vi "AutoRun.vi"() -> ()   [LabVIEW 2012]
uses:
  resultShow.vi
panel:
  in  "布尔":bool
  out "毫秒计时值":u32
  in  "stepMotor/ECU":string
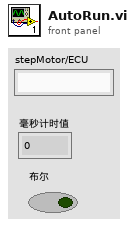
[diagram p1: front panel]
types:
  T1 = cluster{"takesTime":refnum<vi>, "userStatus":refnum<vi>, "userName":refnum<vi>, "connectionMode":refnum<vi>, "productsName":refnum<vi>, "rigStatus":refnum<vi>, "管柱码":refnum<vi>}
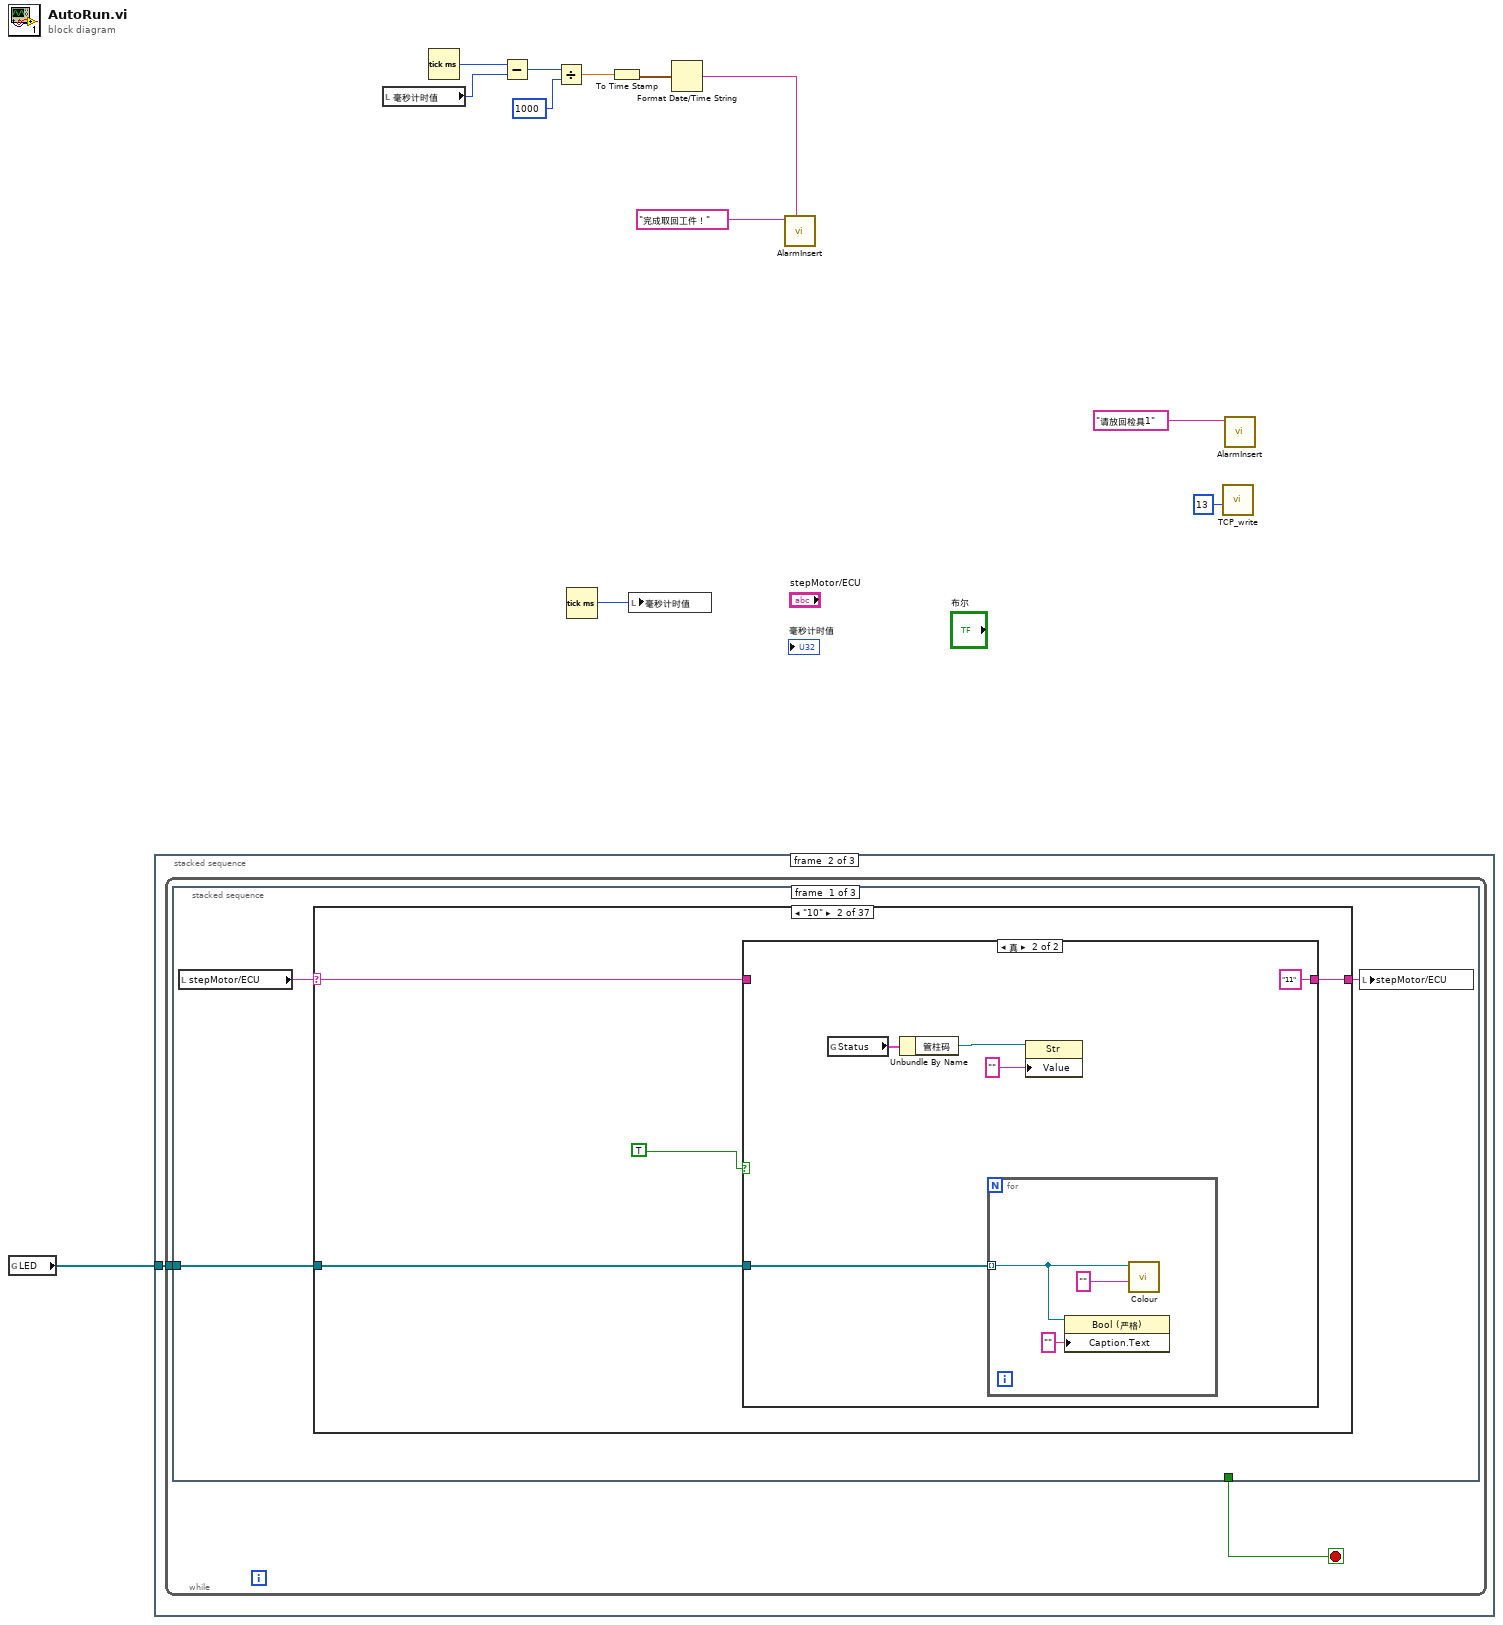
[diagram p0: block diagram]
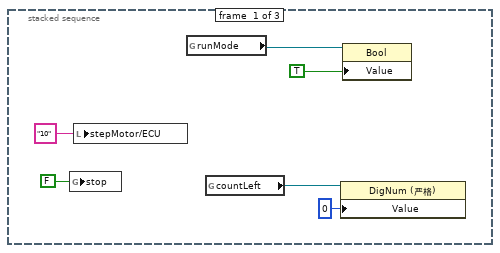
[diagram p2: hidden frame]
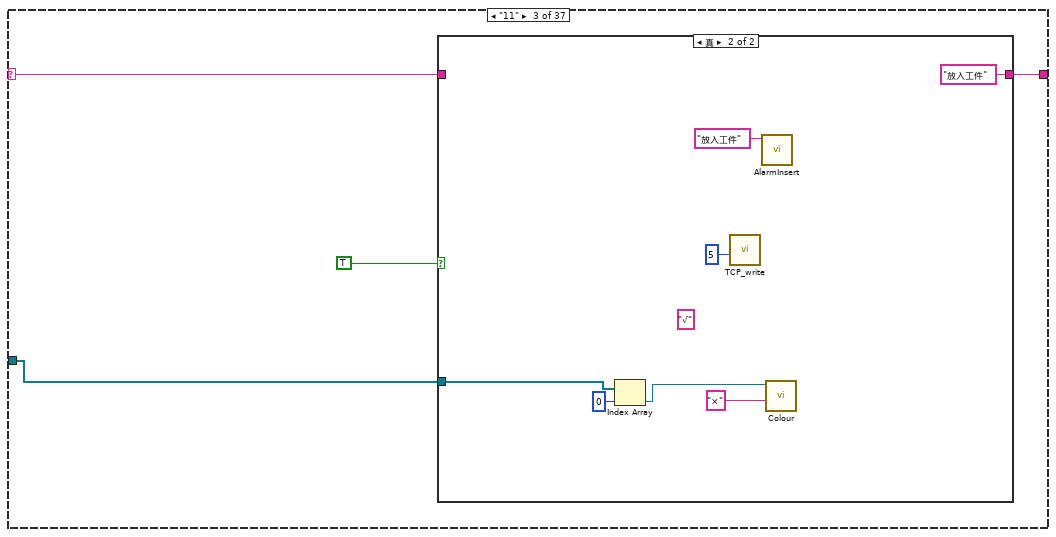
[diagram p5: hidden frame]
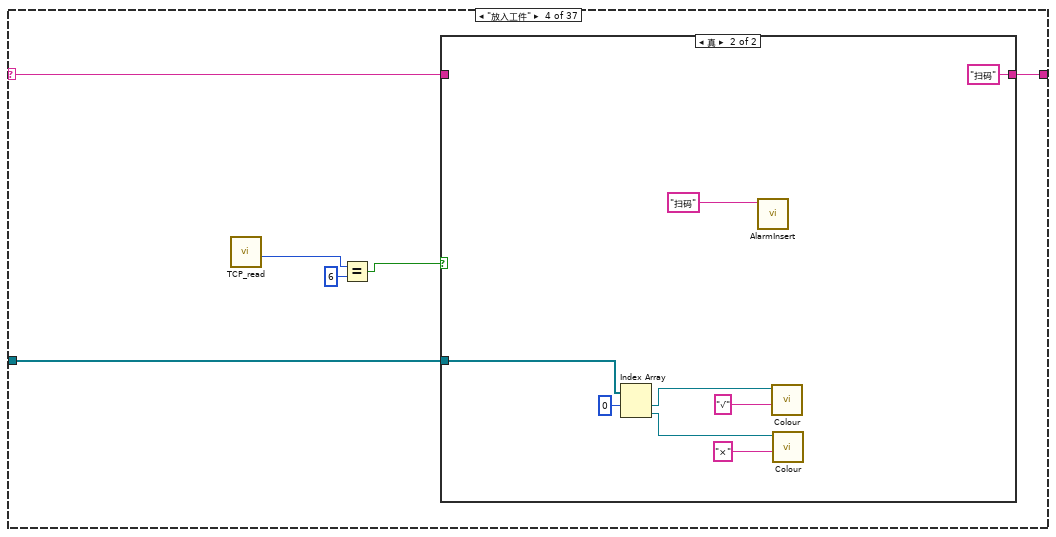
[diagram p7: hidden frame]
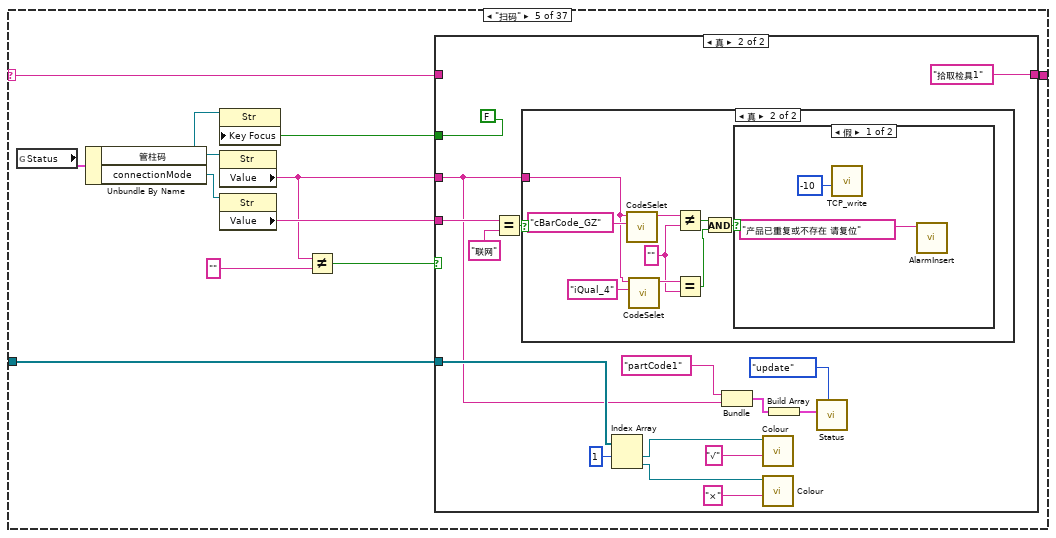
[diagram p9: hidden frame]
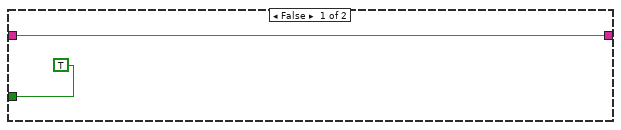
[diagram p10: hidden frame]
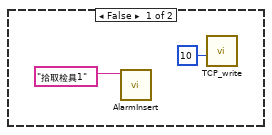
[diagram p11: hidden frame]
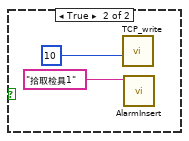
[diagram p12: hidden frame]
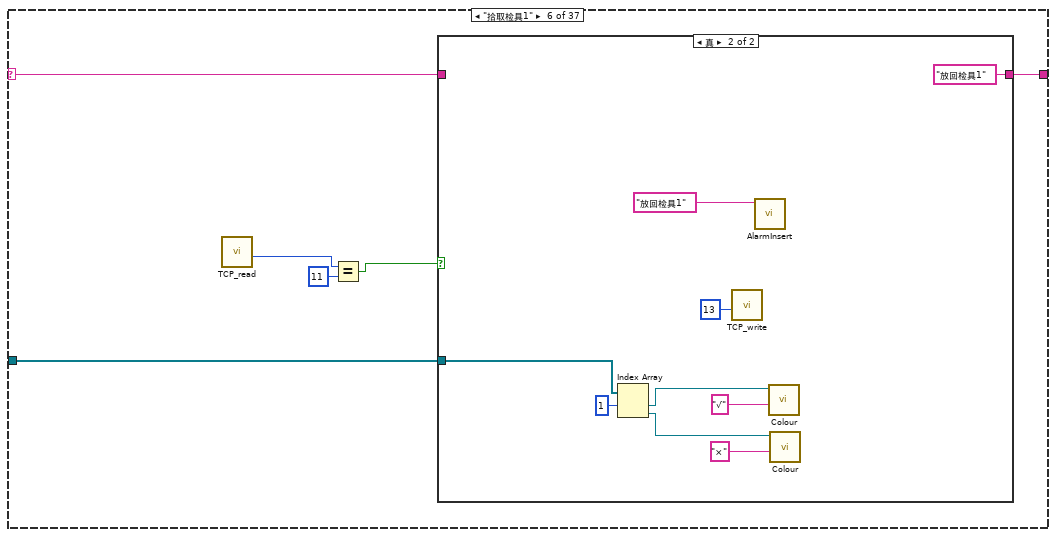
[diagram p13: hidden frame]
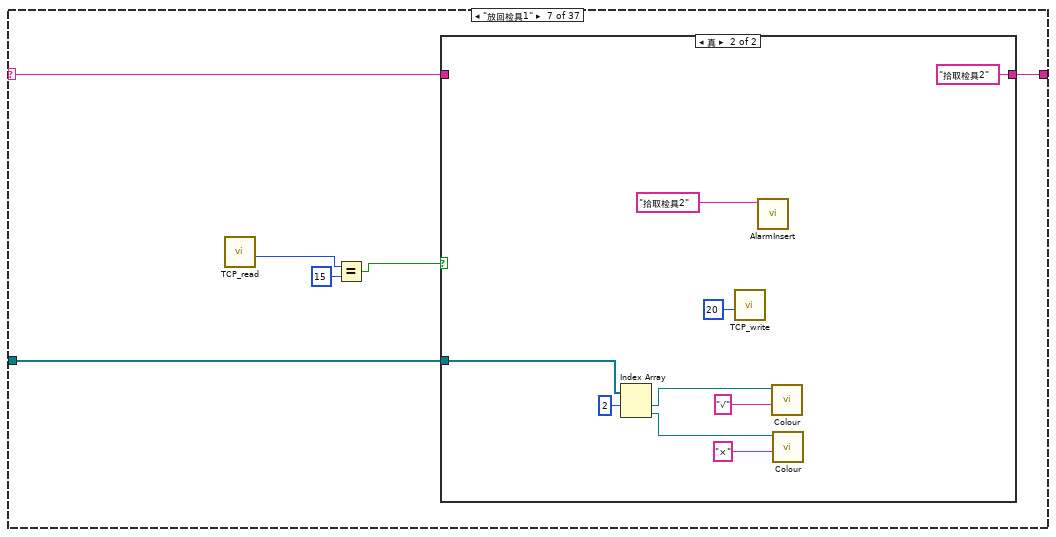
[diagram p15: hidden frame]
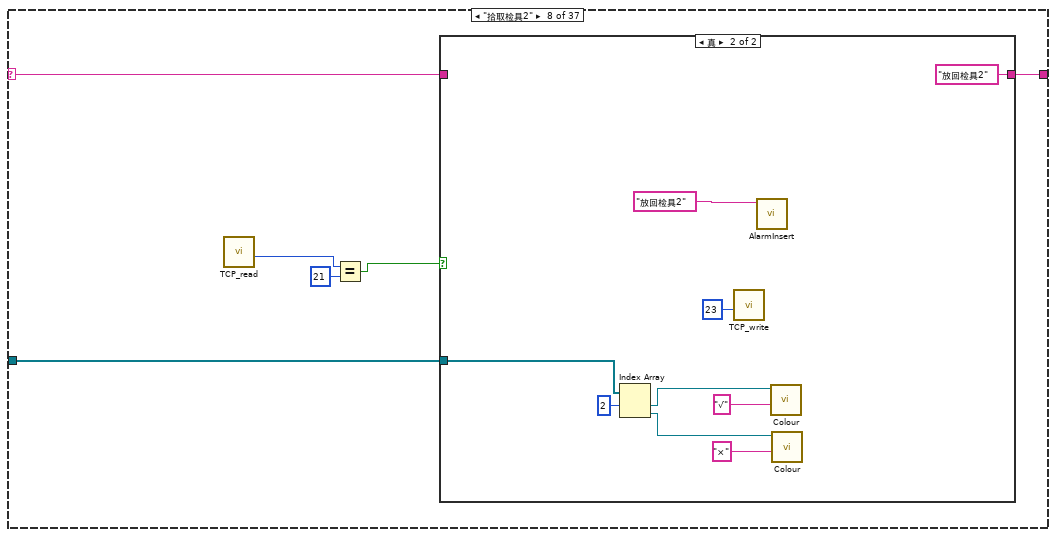
[diagram p17: hidden frame]
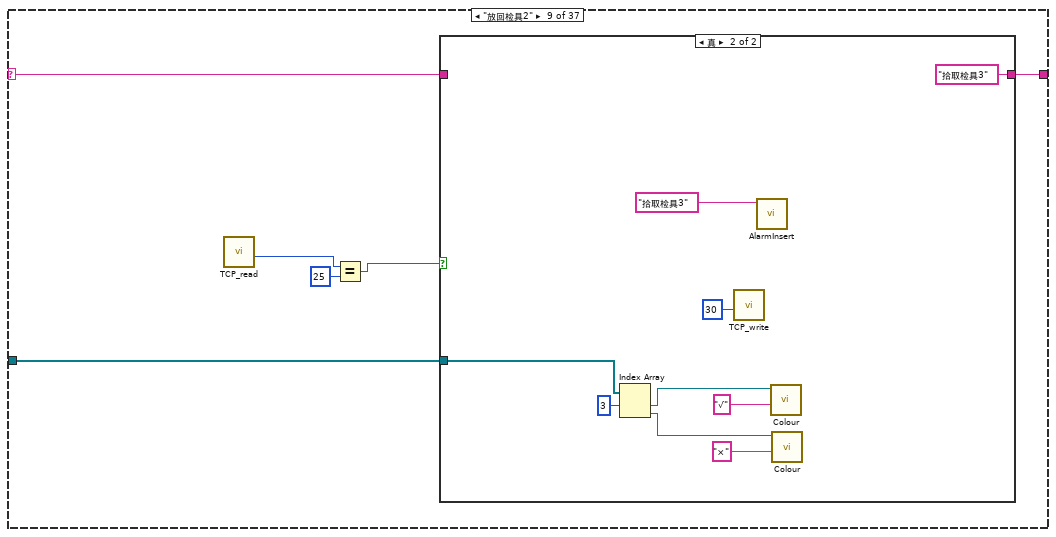
[diagram p19: hidden frame]
diagram:
  n1 = global read "resultShow.vi" "LED"() -> (w12:refnum<vi>[])
  n2 = stacked-sequence {
    tunnel: w12 -> [_ w19 _]
    frame #0 {
      n3 = global write "全局 3.vi" "stop"(FALSE ("布尔 2")) -> ()
      n4 = local write "stepMotor/ECU"("10" ("step")) -> ()
      n5 = global read "resultShow.vi" "runMode"() -> (w15:refnum<vi>)
      n6 = global read "resultShow.vi" "countLeft"() -> (w13:refnum<vi>)
      n7 = property class="DigNum (严格)"(reference=w13, "Value"=u32 0 ("值")) -> ()  [unwired: 1 in, 2 out]
      n8 = property class="Bool"(reference=w15, "Value"=TRUE ("m")) -> ()  [unwired: 1 in, 2 out]
    }
    frame #1 {
      n9 = while {
        tunnel: w19 -> [w20]
        stop <- w21 stop-if-true
        n10 = stacked-sequence {
          tunnel: [_ _ w657] -> w21
          tunnel: w20 -> [w23 _ _]
          frame #0 {
            n11 = local read "stepMotor/ECU"() -> (w22:string)
            n12 = case shown="\"10\"" w22 {
              selector: w22 -> [w25 w28 w41 w53 w75 w114 w128 w144 w160 w178 w194 w210 w226 w242 w258 w274 w290 w306 w322 w338 w354 w370 w386 w402 w418 w434 w450 w466 w482 w498 w514 w530 w546 w562 w578 w592 w620]
              tunnel: [w25 w29 w42 w51 w74 w115 w126 w142 w158 w179 w195 w211 w227 w243 w259 w275 w291 w307 w323 w339 w355 w371 w387 w403 w419 w435 w451 w467 w483 w499 w515 w531 w547 w563 w579 w593 w621] -> w24
              tunnel: w23 -> [_ w27 w40 w52 w76 w110 w127 w143 w159 w174 w190 w206 w222 w238 w254 w270 w286 w302 w318 w334 w350 w366 w382 w398 w414 w430 w446 w462 w478 w494 w510 w526 w542 w558 w574 w591 w616]
              frame "假", Default {
              }
              frame "10" {
                n13 = case shown="真" TRUE {
                  tunnel: [w30 "11"] -> w29
                  tunnel: w28 -> [w30 _]
                  tunnel: w27 -> [_ w34]
                  frame False {
                  }
                  frame True {
                    n14 = global read "resultShow.vi" "Status"() -> (w32:T1)
                    n15 = Unbundle By Name(w32) -> ("管柱码"=w31:refnum<vi>)
                    n16 = for {
                      tunnel: w34 -> [w37] mode=indexing
                      n17 = property class="Bool (严格)"(reference=w37, "Caption.Text"="" ("标题.文本")) -> ()  [unwired: 1 in, 2 out]
                      n18 = call "Colour.vi"("result"="" ("元素"), "colourRef"=w37) -> ()  [unwired: 9 in, 1 out]
                    }
                    n19 = property class="Str"(reference=w31, "Value"="") -> ()  [unwired: 1 in, 2 out]
                  }
                }
              }
              frame "11" {
                n20 = case shown="真" TRUE {
                  tunnel: [w43 "放入工件"] -> w42
                  tunnel: w41 -> [w43 _]
                  tunnel: w40 -> [_ w46]
                  frame False {
                  }
                  frame True {
                    (unwired) "√" ("元素")
                    n21 = Index Array(array=w46, index=0 ("索引")) -> (element=w48:refnum<vi>)
                    n22 = call "TCP_write.vi"("写入数据"=i8 5) -> ()  [unwired: 11 in]
                    n23 = call "AlarmInsert.vi"("消息名"="放入工件") -> ()  [unwired: 11 in]
                    n24 = call "Colour.vi"("result"="×" ("元素"), "colourRef"=w48) -> ()  [unwired: 9 in, 1 out]
                  }
                }
              }
              frame "放入工件" {
                n25 = call "TCP_read.vi"() -> ("元素"=w54:i8)  [unwired: 10 in, 1 out]
                n26 = Equal?(x=w54, y=i8 6) -> (x = y?=w56:bool)
                n27 = case shown="真" w56 {
                  tunnel: [w57 "扫码"] -> w51
                  tunnel: w53 -> [w57 _]
                  tunnel: w52 -> [_ w59]
                  frame False {
                  }
                  frame True {
                    n28 = Index Array(array=w59, index #1=0 ("索引")) -> (element #1=w63:refnum<vi>, element #2=w60:refnum<vi>)  [unwired: 1 in]
                    n29 = call "AlarmInsert.vi"("消息名"="扫码" ("string_5")) -> ()  [unwired: 11 in]
                    n30 = call "Colour.vi"("result"="√" ("元素"), "colourRef"=w63) -> ()  [unwired: 9 in, 1 out]
                    n31 = call "Colour.vi"("result"="×" ("元素"), "colourRef"=w60) -> ()  [unwired: 9 in, 1 out]
                  }
                }
              }
              frame "扫码" {
                n32 = global read "resultShow.vi" "Status"() -> (w73:T1)
                n33 = Unbundle By Name(w73) -> ("管柱码"=w71:refnum<vi>, "connectionMode"=w68:refnum<vi>)
                n34 = property class="Str"(reference=w71) -> ("Value"=w66:string)  [unwired: 1 in, 2 out]
                n35 = property class="Str"(reference=w68) -> ("Value"=w67:string)  [unwired: 1 in, 2 out]
                n36 = Not Equal?(x=w66, y="") -> (x != y?=w70:bool)
                n37 = case shown="真" w70 {
                  tunnel: [w78 "拾取检具1"] -> w74
                  tunnel: w75 -> [w78 _]
                  tunnel: w76 -> [_ w90]
                  tunnel: [TRUE FALSE] -> w69
                  tunnel: w67 -> [_ w85]
                  tunnel: w66 -> [_ w81]
                  frame False {
                  }
                  frame True {
                    n38 = Equal?(x=w85, y="联网") -> (x = y?=w84:bool)
                    n39 = case shown="真" w84 {
                      tunnel: w81 -> [_ w100]
                      frame False {
                        n40 = call "AlarmInsert.vi"("消息名"="拾取检具1") -> ()  [unwired: 11 in]
                        n41 = call "TCP_write.vi"("写入数据"=i8 10) -> ()  [unwired: 11 in]
                      }
                      frame True {
                        w97 = "" ("元素")
                        n42 = call "CodeSelet.vi"("字符串"="cBarCode_GZ" ("code"), "parameter name"=w100) -> ("readData"=w102:string)  [unwired: 9 in]
                        n43 = call "CodeSelet.vi"("字符串"="iQual_4" ("code"), "parameter name"=w100) -> ("readData"=w99:string)  [unwired: 9 in]
                        n44 = Not Equal?(x=w102, y=w97) -> (x != y?=w105:bool)
                        n45 = Equal?(x=w99, y=w97) -> (x = y?=w104:bool)
                        n46 = And(x=w105, y=w104) -> (x .and. y?=w103:bool)
                        n47 = case shown="假" w103 {
                          frame False {
                            n48 = call "TCP_write.vi"("写入数据"=i8 -10) -> ()  [unwired: 11 in]
                            n49 = call "AlarmInsert.vi"("消息名"="产品已重复或不存在 请复位") -> ()  [unwired: 11 in]
                          }
                          frame True {
                            n50 = call "TCP_write.vi"("写入数据"=i8 10) -> ()  [unwired: 11 in]
                            n51 = call "AlarmInsert.vi"("消息名"="拾取检具1") -> ()  [unwired: 11 in]
                          }
                        }
                      }
                    }
                    n52 = Index Array(array=w90, index #1=1 ("索引")) -> (element #1=w92:refnum<vi>, element #2=w88:refnum<vi>)  [unwired: 1 in]
                    n53 = Bundle("元素"="partCode1", "Value"=w81) -> (w83:cluster{"元素":string, "Value":string})  [unwired: 1 in]
                    n54 = call "Colour.vi"("result"="√" ("元素"), "colourRef"=w92) -> ()  [unwired: 9 in, 1 out]
                    n55 = call "Colour.vi"("result"="×" ("元素"), "colourRef"=w88) -> ()  [unwired: 9 in, 1 out]
                    n56 = Build Array(w83) -> (w80:cluster{"元素":string, "Value":string}[])
                    n57 = call "Status.vi"("模式"=enum16{"select", "insert", "update", "delete"}."update", "nameData"=w80) -> ()  [unwired: 9 in, 1 out]
                  }
                }
                n58 = property class="Str"(reference=w71, "Key Focus"=w69) -> ()  [unwired: 1 in, 2 out]
              }
              frame "拾取检具1" {
                n59 = call "TCP_read.vi"() -> ("元素"=w113:i8)  [unwired: 10 in, 1 out]
                n60 = Equal?(x=w113, y=i8 11) -> (x = y?=w111:bool)
                n61 = case shown="真" w111 {
                  tunnel: [w116 "放回检具1"] -> w115
                  tunnel: w114 -> [w116 _]
                  tunnel: w110 -> [_ w118]
                  frame False {
                  }
                  frame True {
                    n62 = Index Array(array=w118, index #1=1 ("索引")) -> (element #1=w122:refnum<vi>, element #2=w119:refnum<vi>)  [unwired: 1 in]
                    n63 = call "TCP_write.vi"("写入数据"=i8 13) -> ()  [unwired: 11 in]
                    n64 = call "AlarmInsert.vi"("消息名"="放回检具1" ("string_5")) -> ()  [unwired: 11 in]
                    n65 = call "Colour.vi"("result"="√" ("元素"), "colourRef"=w122) -> ()  [unwired: 9 in, 1 out]
                    n66 = call "Colour.vi"("result"="×" ("元素"), "colourRef"=w119) -> ()  [unwired: 9 in, 1 out]
                  }
                }
              }
              frame "放回检具1" {
                n67 = call "TCP_read.vi"() -> ("元素"=w131:i8)  [unwired: 10 in, 1 out]
                n68 = Equal?(x=w131, y=i8 15) -> (x = y?=w129:bool)
                n69 = case shown="真" w129 {
                  tunnel: [w132 "拾取检具2"] -> w126
                  tunnel: w128 -> [w132 _]
                  tunnel: w127 -> [_ w134]
                  frame False {
                  }
                  frame True {
                    n70 = Index Array(array=w134, index #1=2 ("索引")) -> (element #1=w138:refnum<vi>, element #2=w135:refnum<vi>)  [unwired: 1 in]
                    n71 = call "TCP_write.vi"("写入数据"=i8 20) -> ()  [unwired: 11 in]
                    n72 = call "AlarmInsert.vi"("消息名"="拾取检具2" ("string_5")) -> ()  [unwired: 11 in]
                    n73 = call "Colour.vi"("result"="√" ("元素"), "colourRef"=w138) -> ()  [unwired: 9 in, 1 out]
                    n74 = call "Colour.vi"("result"="×" ("元素"), "colourRef"=w135) -> ()  [unwired: 9 in, 1 out]
                  }
                }
              }
              frame "拾取检具2" {
                n75 = call "TCP_read.vi"() -> ("元素"=w145:i8)  [unwired: 10 in, 1 out]
                n76 = Equal?(x=w145, y=i8 21) -> (x = y?=w147:bool)
                n77 = case shown="真" w147 {
                  tunnel: [w148 "放回检具2"] -> w142
                  tunnel: w144 -> [w148 _]
                  tunnel: w143 -> [_ w150]
                  frame False {
                  }
                  frame True {
                    n78 = Index Array(array=w150, index #1=2 ("索引")) -> (element #1=w154:refnum<vi>, element #2=w151:refnum<vi>)  [unwired: 1 in]
                    n79 = call "TCP_write.vi"("写入数据"=i8 23) -> ()  [unwired: 11 in]
                    n80 = call "AlarmInsert.vi"("消息名"="放回检具2" ("string_5")) -> ()  [unwired: 11 in]
                    n81 = call "Colour.vi"("result"="√" ("元素"), "colourRef"=w154) -> ()  [unwired: 9 in, 1 out]
                    n82 = call "Colour.vi"("result"="×" ("元素"), "colourRef"=w151) -> ()  [unwired: 9 in, 1 out]
                  }
                }
              }
              frame "放回检具2" {
                n83 = call "TCP_read.vi"() -> ("元素"=w161:i8)  [unwired: 10 in, 1 out]
                n84 = Equal?(x=w161, y=i8 25) -> (x = y?=w163:bool)
                n85 = case shown="真" w163 {
                  tunnel: [w164 "拾取检具3"] -> w158
                  tunnel: w160 -> [w164 _]
                  tunnel: w159 -> [_ w166]
                  frame False {
                  }
                  frame True {
                    n86 = Index Array(array=w166, index #1=3 ("索引")) -> (element #1=w170:refnum<vi>, element #2=w167:refnum<vi>)  [unwired: 1 in]
                    n87 = call "TCP_write.vi"("写入数据"=i8 30) -> ()  [unwired: 11 in]
                    n88 = call "AlarmInsert.vi"("消息名"="拾取检具3" ("string_5")) -> ()  [unwired: 11 in]
                    n89 = call "Colour.vi"("result"="√" ("元素"), "colourRef"=w170) -> ()  [unwired: 9 in, 1 out]
                    n90 = call "Colour.vi"("result"="×" ("元素"), "colourRef"=w167) -> ()  [unwired: 9 in, 1 out]
                  }
                }
              }
              frame "拾取检具3" {
                n91 = call "TCP_read.vi"() -> ("元素"=w177:i8)  [unwired: 10 in, 1 out]
                n92 = Equal?(x=w177, y=i8 31) -> (x = y?=w175:bool)
                n93 = case shown="真" w175 {
                  tunnel: [w180 "放回检具3"] -> w179
                  tunnel: w178 -> [w180 _]
                  tunnel: w174 -> [_ w182]
                  frame False {
                  }
                  frame True {
                    n94 = Index Array(array=w182, index #1=3 ("索引")) -> (element #1=w186:refnum<vi>, element #2=w183:refnum<vi>)  [unwired: 1 in]
                    n95 = call "TCP_write.vi"("写入数据"=i8 33) -> ()  [unwired: 11 in]
                    n96 = call "AlarmInsert.vi"("消息名"="放回检具3" ("string_5")) -> ()  [unwired: 11 in]
                    n97 = call "Colour.vi"("result"="√" ("元素"), "colourRef"=w186) -> ()  [unwired: 9 in, 1 out]
                    n98 = call "Colour.vi"("result"="×" ("元素"), "colourRef"=w183) -> ()  [unwired: 9 in, 1 out]
                  }
                }
              }
              frame "放回检具3" {
                n99 = call "TCP_read.vi"() -> ("元素"=w193:i8)  [unwired: 10 in, 1 out]
                n100 = Equal?(x=w193, y=i8 35) -> (x = y?=w191:bool)
                n101 = case shown="真" w191 {
                  tunnel: [w196 "拾取检具4"] -> w195
                  tunnel: w194 -> [w196 _]
                  tunnel: w190 -> [_ w198]
                  frame False {
                  }
                  frame True {
                    n102 = Index Array(array=w198, index #1=4 ("索引")) -> (element #1=w202:refnum<vi>, element #2=w199:refnum<vi>)  [unwired: 1 in]
                    n103 = call "TCP_write.vi"("写入数据"=i8 40) -> ()  [unwired: 11 in]
                    n104 = call "AlarmInsert.vi"("消息名"="拾取检具4" ("string_5")) -> ()  [unwired: 11 in]
                    n105 = call "Colour.vi"("result"="√" ("元素"), "colourRef"=w202) -> ()  [unwired: 9 in, 1 out]
                    n106 = call "Colour.vi"("result"="×" ("元素"), "colourRef"=w199) -> ()  [unwired: 9 in, 1 out]
                  }
                }
              }
              frame "拾取检具4" {
                n107 = call "TCP_read.vi"() -> ("元素"=w209:i8)  [unwired: 10 in, 1 out]
                n108 = Equal?(x=w209, y=i8 41) -> (x = y?=w207:bool)
                n109 = case shown="真" w207 {
                  tunnel: [w212 "放回检具4"] -> w211
                  tunnel: w210 -> [w212 _]
                  tunnel: w206 -> [_ w214]
                  frame False {
                  }
                  frame True {
                    n110 = Index Array(array=w214, index #1=4 ("索引")) -> (element #1=w218:refnum<vi>, element #2=w215:refnum<vi>)  [unwired: 1 in]
                    n111 = call "TCP_write.vi"("写入数据"=i8 43) -> ()  [unwired: 11 in]
                    n112 = call "AlarmInsert.vi"("消息名"="放回检具4" ("string_5")) -> ()  [unwired: 11 in]
                    n113 = call "Colour.vi"("result"="√" ("元素"), "colourRef"=w218) -> ()  [unwired: 9 in, 1 out]
                    n114 = call "Colour.vi"("result"="×" ("元素"), "colourRef"=w215) -> ()  [unwired: 9 in, 1 out]
                  }
                }
              }
              frame "放回检具4" {
                n115 = call "TCP_read.vi"() -> ("元素"=w225:i8)  [unwired: 10 in, 1 out]
                n116 = Equal?(x=w225, y=i8 45) -> (x = y?=w223:bool)
                n117 = case shown="真" w223 {
                  tunnel: [w228 "拾取检具5"] -> w227
                  tunnel: w226 -> [w228 _]
                  tunnel: w222 -> [_ w230]
                  frame False {
                  }
                  frame True {
                    n118 = Index Array(array=w230, index #1=5 ("索引")) -> (element #1=w234:refnum<vi>, element #2=w231:refnum<vi>)  [unwired: 1 in]
                    n119 = call "TCP_write.vi"("写入数据"=i8 50) -> ()  [unwired: 11 in]
                    n120 = call "AlarmInsert.vi"("消息名"="拾取检具5" ("string_5")) -> ()  [unwired: 11 in]
                    n121 = call "Colour.vi"("result"="√" ("元素"), "colourRef"=w234) -> ()  [unwired: 9 in, 1 out]
                    n122 = call "Colour.vi"("result"="×" ("元素"), "colourRef"=w231) -> ()  [unwired: 9 in, 1 out]
                  }
                }
              }
              frame "拾取检具5" {
                n123 = call "TCP_read.vi"() -> ("元素"=w241:i8)  [unwired: 10 in, 1 out]
                n124 = Equal?(x=w241, y=i8 51) -> (x = y?=w239:bool)
                n125 = case shown="真" w239 {
                  tunnel: [w244 "放回检具5"] -> w243
                  tunnel: w242 -> [w244 _]
                  tunnel: w238 -> [_ w246]
                  frame False {
                  }
                  frame True {
                    n126 = Index Array(array=w246, index #1=5 ("索引")) -> (element #1=w250:refnum<vi>, element #2=w247:refnum<vi>)  [unwired: 1 in]
                    n127 = call "TCP_write.vi"("写入数据"=i8 53) -> ()  [unwired: 11 in]
                    n128 = call "AlarmInsert.vi"("消息名"="放回检具5" ("string_5")) -> ()  [unwired: 11 in]
                    n129 = call "Colour.vi"("result"="√" ("元素"), "colourRef"=w250) -> ()  [unwired: 9 in, 1 out]
                    n130 = call "Colour.vi"("result"="×" ("元素"), "colourRef"=w247) -> ()  [unwired: 9 in, 1 out]
                  }
                }
              }
              frame "放回检具5" {
                n131 = call "TCP_read.vi"() -> ("元素"=w257:i8)  [unwired: 10 in, 1 out]
                n132 = Equal?(x=w257, y=i8 55) -> (x = y?=w255:bool)
                n133 = case shown="真" w255 {
                  tunnel: [w260 "拾取检具6"] -> w259
                  tunnel: w258 -> [w260 _]
                  tunnel: w254 -> [_ w262]
                  frame False {
                  }
                  frame True {
                    n134 = Index Array(array=w262, index #1=6 ("索引")) -> (element #1=w266:refnum<vi>, element #2=w263:refnum<vi>)  [unwired: 1 in]
                    n135 = call "TCP_write.vi"("写入数据"=i8 60) -> ()  [unwired: 11 in]
                    n136 = call "AlarmInsert.vi"("消息名"="拾取检具6" ("string_5")) -> ()  [unwired: 11 in]
                    n137 = call "Colour.vi"("result"="√" ("元素"), "colourRef"=w266) -> ()  [unwired: 9 in, 1 out]
                    n138 = call "Colour.vi"("result"="×" ("元素"), "colourRef"=w263) -> ()  [unwired: 9 in, 1 out]
                  }
                }
              }
              frame "拾取检具6" {
                n139 = call "TCP_read.vi"() -> ("元素"=w273:i8)  [unwired: 10 in, 1 out]
                n140 = Equal?(x=w273, y=i8 61) -> (x = y?=w271:bool)
                n141 = case shown="真" w271 {
                  tunnel: [w276 "放回检具6"] -> w275
                  tunnel: w274 -> [w276 _]
                  tunnel: w270 -> [_ w278]
                  frame False {
                  }
                  frame True {
                    n142 = Index Array(array=w278, index #1=6 ("索引")) -> (element #1=w282:refnum<vi>, element #2=w279:refnum<vi>)  [unwired: 1 in]
                    n143 = call "TCP_write.vi"("写入数据"=i8 63) -> ()  [unwired: 11 in]
                    n144 = call "AlarmInsert.vi"("消息名"="放回检具6" ("string_5")) -> ()  [unwired: 11 in]
                    n145 = call "Colour.vi"("result"="√" ("元素"), "colourRef"=w282) -> ()  [unwired: 9 in, 1 out]
                    n146 = call "Colour.vi"("result"="×" ("元素"), "colourRef"=w279) -> ()  [unwired: 9 in, 1 out]
                  }
                }
              }
              frame "放回检具6" {
                n147 = call "TCP_read.vi"() -> ("元素"=w289:i8)  [unwired: 10 in, 1 out]
                n148 = Equal?(x=w289, y=i8 65) -> (x = y?=w287:bool)
                n149 = case shown="真" w287 {
                  tunnel: [w292 "拾取检具7"] -> w291
                  tunnel: w290 -> [w292 _]
                  tunnel: w286 -> [_ w294]
                  frame False {
                  }
                  frame True {
                    n150 = Index Array(array=w294, index #1=7 ("索引")) -> (element #1=w298:refnum<vi>, element #2=w295:refnum<vi>)  [unwired: 1 in]
                    n151 = call "TCP_write.vi"("写入数据"=i8 70) -> ()  [unwired: 11 in]
                    n152 = call "AlarmInsert.vi"("消息名"="拾取检具7" ("string_5")) -> ()  [unwired: 11 in]
                    n153 = call "Colour.vi"("result"="√" ("元素"), "colourRef"=w298) -> ()  [unwired: 9 in, 1 out]
                    n154 = call "Colour.vi"("result"="×" ("元素"), "colourRef"=w295) -> ()  [unwired: 9 in, 1 out]
                  }
                }
              }
              frame "拾取检具7" {
                n155 = call "TCP_read.vi"() -> ("元素"=w305:i8)  [unwired: 10 in, 1 out]
                n156 = Equal?(x=w305, y=i8 71) -> (x = y?=w303:bool)
                n157 = case shown="真" w303 {
                  tunnel: [w308 "放回检具7"] -> w307
                  tunnel: w306 -> [w308 _]
                  tunnel: w302 -> [_ w310]
                  frame False {
                  }
                  frame True {
                    n158 = Index Array(array=w310, index #1=7 ("索引")) -> (element #1=w314:refnum<vi>, element #2=w311:refnum<vi>)  [unwired: 1 in]
                    n159 = call "TCP_write.vi"("写入数据"=i8 73) -> ()  [unwired: 11 in]
                    n160 = call "AlarmInsert.vi"("消息名"="放回检具7" ("string_5")) -> ()  [unwired: 11 in]
                    n161 = call "Colour.vi"("result"="√" ("元素"), "colourRef"=w314) -> ()  [unwired: 9 in, 1 out]
                    n162 = call "Colour.vi"("result"="×" ("元素"), "colourRef"=w311) -> ()  [unwired: 9 in, 1 out]
                  }
                }
              }
              frame "放回检具7" {
                n163 = call "TCP_read.vi"() -> ("元素"=w321:i8)  [unwired: 10 in, 1 out]
                n164 = Equal?(x=w321, y=i8 75) -> (x = y?=w319:bool)
                n165 = case shown="真" w319 {
                  tunnel: [w324 "拾取检具8"] -> w323
                  tunnel: w322 -> [w324 _]
                  tunnel: w318 -> [_ w326]
                  frame False {
                  }
                  frame True {
                    n166 = Index Array(array=w326, index #1=8 ("索引")) -> (element #1=w330:refnum<vi>, element #2=w327:refnum<vi>)  [unwired: 1 in]
                    n167 = call "TCP_write.vi"("写入数据"=i8 80) -> ()  [unwired: 11 in]
                    n168 = call "AlarmInsert.vi"("消息名"="拾取检具8" ("string_5")) -> ()  [unwired: 11 in]
                    n169 = call "Colour.vi"("result"="√" ("元素"), "colourRef"=w330) -> ()  [unwired: 9 in, 1 out]
                    n170 = call "Colour.vi"("result"="×" ("元素"), "colourRef"=w327) -> ()  [unwired: 9 in, 1 out]
                  }
                }
              }
              frame "拾取检具8" {
                n171 = call "TCP_read.vi"() -> ("元素"=w337:i8)  [unwired: 10 in, 1 out]
                n172 = Equal?(x=w337, y=i8 81) -> (x = y?=w335:bool)
                n173 = case shown="真" w335 {
                  tunnel: [w340 "放回检具8"] -> w339
                  tunnel: w338 -> [w340 _]
                  tunnel: w334 -> [_ w342]
                  frame False {
                  }
                  frame True {
                    n174 = Index Array(array=w342, index #1=8 ("索引")) -> (element #1=w346:refnum<vi>, element #2=w343:refnum<vi>)  [unwired: 1 in]
                    n175 = call "TCP_write.vi"("写入数据"=i8 83) -> ()  [unwired: 11 in]
                    n176 = call "AlarmInsert.vi"("消息名"="放回检具8" ("string_5")) -> ()  [unwired: 11 in]
                    n177 = call "Colour.vi"("result"="√" ("元素"), "colourRef"=w346) -> ()  [unwired: 9 in, 1 out]
                    n178 = call "Colour.vi"("result"="×" ("元素"), "colourRef"=w343) -> ()  [unwired: 9 in, 1 out]
                  }
                }
              }
              frame "放回检具8" {
                n179 = call "TCP_read.vi"() -> ("元素"=w353:i8)  [unwired: 10 in, 1 out]
                n180 = Equal?(x=w353, y=i8 85) -> (x = y?=w351:bool)
                n181 = case shown="真" w351 {
                  tunnel: [w356 "拾取检具9"] -> w355
                  tunnel: w354 -> [w356 _]
                  tunnel: w350 -> [_ w358]
                  frame False {
                  }
                  frame True {
                    n182 = Index Array(array=w358, index #1=9 ("索引")) -> (element #1=w362:refnum<vi>, element #2=w359:refnum<vi>)  [unwired: 1 in]
                    n183 = call "TCP_write.vi"("写入数据"=i8 86) -> ()  [unwired: 11 in]
                    n184 = call "AlarmInsert.vi"("消息名"="拾取检具9" ("string_5")) -> ()  [unwired: 11 in]
                    n185 = call "Colour.vi"("result"="√" ("元素"), "colourRef"=w362) -> ()  [unwired: 9 in, 1 out]
                    n186 = call "Colour.vi"("result"="×" ("元素"), "colourRef"=w359) -> ()  [unwired: 9 in, 1 out]
                  }
                }
              }
              frame "拾取检具9" {
                n187 = call "TCP_read.vi"() -> ("元素"=w369:i8)  [unwired: 10 in, 1 out]
                n188 = Equal?(x=w369, y=i8 87) -> (x = y?=w367:bool)
                n189 = case shown="真" w367 {
                  tunnel: [w372 "放回检具9"] -> w371
                  tunnel: w370 -> [w372 _]
                  tunnel: w366 -> [_ w374]
                  frame False {
                  }
                  frame True {
                    n190 = Index Array(array=w374, index #1=9 ("索引")) -> (element #1=w378:refnum<vi>, element #2=w375:refnum<vi>)  [unwired: 1 in]
                    n191 = call "TCP_write.vi"("写入数据"=i8 88) -> ()  [unwired: 11 in]
                    n192 = call "AlarmInsert.vi"("消息名"="放回检具9" ("string_5")) -> ()  [unwired: 11 in]
                    n193 = call "Colour.vi"("result"="√" ("元素"), "colourRef"=w378) -> ()  [unwired: 9 in, 1 out]
                    n194 = call "Colour.vi"("result"="×" ("元素"), "colourRef"=w375) -> ()  [unwired: 9 in, 1 out]
                  }
                }
              }
              frame "放回检具9" {
                n195 = call "TCP_read.vi"() -> ("元素"=w385:i8)  [unwired: 10 in, 1 out]
                n196 = Equal?(x=w385, y=i8 89) -> (x = y?=w383:bool)
                n197 = case shown="真" w383 {
                  tunnel: [w388 "拾取检具10"] -> w387
                  tunnel: w386 -> [w388 _]
                  tunnel: w382 -> [_ w390]
                  frame False {
                  }
                  frame True {
                    n198 = Index Array(array=w390, index #1=10 ("索引")) -> (element #1=w394:refnum<vi>, element #2=w391:refnum<vi>)  [unwired: 1 in]
                    n199 = call "TCP_write.vi"("写入数据"=i8 90) -> ()  [unwired: 11 in]
                    n200 = call "AlarmInsert.vi"("消息名"="拾取检具10" ("string_5")) -> ()  [unwired: 11 in]
                    n201 = call "Colour.vi"("result"="√" ("元素"), "colourRef"=w394) -> ()  [unwired: 9 in, 1 out]
                    n202 = call "Colour.vi"("result"="×" ("元素"), "colourRef"=w391) -> ()  [unwired: 9 in, 1 out]
                  }
                }
              }
              frame "拾取检具10" {
                n203 = call "TCP_read.vi"() -> ("元素"=w401:i8)  [unwired: 10 in, 1 out]
                n204 = Equal?(x=w401, y=i8 91) -> (x = y?=w399:bool)
                n205 = case shown="真" w399 {
                  tunnel: [w404 "放回检具10"] -> w403
                  tunnel: w402 -> [w404 _]
                  tunnel: w398 -> [_ w406]
                  frame False {
                  }
                  frame True {
                    n206 = Index Array(array=w406, index #1=10 ("索引")) -> (element #1=w410:refnum<vi>, element #2=w407:refnum<vi>)  [unwired: 1 in]
                    n207 = call "TCP_write.vi"("写入数据"=i8 92) -> ()  [unwired: 11 in]
                    n208 = call "AlarmInsert.vi"("消息名"="放回检具10" ("string_5")) -> ()  [unwired: 11 in]
                    n209 = call "Colour.vi"("result"="√" ("元素"), "colourRef"=w410) -> ()  [unwired: 9 in, 1 out]
                    n210 = call "Colour.vi"("result"="×" ("元素"), "colourRef"=w407) -> ()  [unwired: 9 in, 1 out]
                  }
                }
              }
              frame "放回检具10" {
                n211 = call "TCP_read.vi"() -> ("元素"=w417:i8)  [unwired: 10 in, 1 out]
                n212 = Equal?(x=w417, y=i8 93) -> (x = y?=w415:bool)
                n213 = case shown="真" w415 {
                  tunnel: [w420 "拾取检具11"] -> w419
                  tunnel: w418 -> [w420 _]
                  tunnel: w414 -> [_ w422]
                  frame False {
                  }
                  frame True {
                    n214 = Index Array(array=w422, index #1=11 ("索引")) -> (element #1=w426:refnum<vi>, element #2=w423:refnum<vi>)  [unwired: 1 in]
                    n215 = call "TCP_write.vi"("写入数据"=i8 94) -> ()  [unwired: 11 in]
                    n216 = call "AlarmInsert.vi"("消息名"="拾取检具11" ("string_5")) -> ()  [unwired: 11 in]
                    n217 = call "Colour.vi"("result"="√" ("元素"), "colourRef"=w426) -> ()  [unwired: 9 in, 1 out]
                    n218 = call "Colour.vi"("result"="×" ("元素"), "colourRef"=w423) -> ()  [unwired: 9 in, 1 out]
                  }
                }
              }
              frame "拾取检具11" {
                n219 = call "TCP_read.vi"() -> ("元素"=w433:i8)  [unwired: 10 in, 1 out]
                n220 = Equal?(x=w433, y=i8 95) -> (x = y?=w431:bool)
                n221 = case shown="真" w431 {
                  tunnel: [w436 "放回检具11"] -> w435
                  tunnel: w434 -> [w436 _]
                  tunnel: w430 -> [_ w438]
                  frame False {
                  }
                  frame True {
                    n222 = Index Array(array=w438, index #1=11 ("索引")) -> (element #1=w442:refnum<vi>, element #2=w439:refnum<vi>)  [unwired: 1 in]
                    n223 = call "TCP_write.vi"("写入数据"=i8 96) -> ()  [unwired: 11 in]
                    n224 = call "AlarmInsert.vi"("消息名"="放回检具11" ("string_5")) -> ()  [unwired: 11 in]
                    n225 = call "Colour.vi"("result"="√" ("元素"), "colourRef"=w442) -> ()  [unwired: 9 in, 1 out]
                    n226 = call "Colour.vi"("result"="×" ("元素"), "colourRef"=w439) -> ()  [unwired: 9 in, 1 out]
                  }
                }
              }
              frame "放回检具11" {
                n227 = call "TCP_read.vi"() -> ("元素"=w449:i8)  [unwired: 10 in, 1 out]
                n228 = Equal?(x=w449, y=i8 97) -> (x = y?=w447:bool)
                n229 = case shown="真" w447 {
                  tunnel: [w452 "拾取检具12"] -> w451
                  tunnel: w450 -> [w452 _]
                  tunnel: w446 -> [_ w454]
                  frame False {
                  }
                  frame True {
                    n230 = Index Array(array=w454, index #1=12 ("索引")) -> (element #1=w458:refnum<vi>, element #2=w455:refnum<vi>)  [unwired: 1 in]
                    n231 = call "TCP_write.vi"("写入数据"=i8 98) -> ()  [unwired: 11 in]
                    n232 = call "AlarmInsert.vi"("消息名"="拾取检具12" ("string_5")) -> ()  [unwired: 11 in]
                    n233 = call "Colour.vi"("result"="√" ("元素"), "colourRef"=w458) -> ()  [unwired: 9 in, 1 out]
                    n234 = call "Colour.vi"("result"="×" ("元素"), "colourRef"=w455) -> ()  [unwired: 9 in, 1 out]
                  }
                }
              }
              frame "拾取检具12" {
                n235 = call "TCP_read.vi"() -> ("元素"=w465:i8)  [unwired: 10 in, 1 out]
                n236 = Equal?(x=w465, y=i8 99) -> (x = y?=w463:bool)
                n237 = case shown="真" w463 {
                  tunnel: [w468 "放回检具12"] -> w467
                  tunnel: w466 -> [w468 _]
                  tunnel: w462 -> [_ w470]
                  frame False {
                  }
                  frame True {
                    n238 = Index Array(array=w470, index #1=12 ("索引")) -> (element #1=w474:refnum<vi>, element #2=w471:refnum<vi>)  [unwired: 1 in]
                    n239 = call "TCP_write.vi"("写入数据"=i8 100) -> ()  [unwired: 11 in]
                    n240 = call "AlarmInsert.vi"("消息名"="放回检具12" ("string_5")) -> ()  [unwired: 11 in]
                    n241 = call "Colour.vi"("result"="√" ("元素"), "colourRef"=w474) -> ()  [unwired: 9 in, 1 out]
                    n242 = call "Colour.vi"("result"="×" ("元素"), "colourRef"=w471) -> ()  [unwired: 9 in, 1 out]
                  }
                }
              }
              frame "放回检具12" {
                n243 = call "TCP_read.vi"() -> ("元素"=w481:i8)  [unwired: 10 in, 1 out]
                n244 = Equal?(x=w481, y=i8 101) -> (x = y?=w479:bool)
                n245 = case shown="真" w479 {
                  tunnel: [w484 "拾取检具13"] -> w483
                  tunnel: w482 -> [w484 _]
                  tunnel: w478 -> [_ w486]
                  frame False {
                  }
                  frame True {
                    n246 = Index Array(array=w486, index #1=13 ("索引")) -> (element #1=w490:refnum<vi>, element #2=w487:refnum<vi>)  [unwired: 1 in]
                    n247 = call "TCP_write.vi"("写入数据"=i8 102) -> ()  [unwired: 11 in]
                    n248 = call "AlarmInsert.vi"("消息名"="拾取检具13" ("string_5")) -> ()  [unwired: 11 in]
                    n249 = call "Colour.vi"("result"="√" ("元素"), "colourRef"=w490) -> ()  [unwired: 9 in, 1 out]
                    n250 = call "Colour.vi"("result"="×" ("元素"), "colourRef"=w487) -> ()  [unwired: 9 in, 1 out]
                  }
                }
              }
              frame "拾取检具13" {
                n251 = call "TCP_read.vi"() -> ("元素"=w497:i8)  [unwired: 10 in, 1 out]
                n252 = Equal?(x=w497, y=i8 103) -> (x = y?=w495:bool)
                n253 = case shown="真" w495 {
                  tunnel: [w500 "放回检具13"] -> w499
                  tunnel: w498 -> [w500 _]
                  tunnel: w494 -> [_ w502]
                  frame False {
                  }
                  frame True {
                    n254 = Index Array(array=w502, index #1=13 ("索引")) -> (element #1=w506:refnum<vi>, element #2=w503:refnum<vi>)  [unwired: 1 in]
                    n255 = call "TCP_write.vi"("写入数据"=i8 104) -> ()  [unwired: 11 in]
                    n256 = call "AlarmInsert.vi"("消息名"="放回检具13" ("string_5")) -> ()  [unwired: 11 in]
                    n257 = call "Colour.vi"("result"="√" ("元素"), "colourRef"=w506) -> ()  [unwired: 9 in, 1 out]
                    n258 = call "Colour.vi"("result"="×" ("元素"), "colourRef"=w503) -> ()  [unwired: 9 in, 1 out]
                  }
                }
              }
              frame "放回检具13" {
                n259 = call "TCP_read.vi"() -> ("元素"=w513:i8)  [unwired: 10 in, 1 out]
                n260 = Equal?(x=w513, y=i8 105) -> (x = y?=w511:bool)
                n261 = case shown="真" w511 {
                  tunnel: [w516 "拾取检具14"] -> w515
                  tunnel: w514 -> [w516 _]
                  tunnel: w510 -> [_ w518]
                  frame False {
                  }
                  frame True {
                    n262 = Index Array(array=w518, index #1=14 ("索引")) -> (element #1=w522:refnum<vi>, element #2=w519:refnum<vi>)  [unwired: 1 in]
                    n263 = call "TCP_write.vi"("写入数据"=i8 106) -> ()  [unwired: 11 in]
                    n264 = call "AlarmInsert.vi"("消息名"="拾取检具14" ("string_5")) -> ()  [unwired: 11 in]
                    n265 = call "Colour.vi"("result"="√" ("元素"), "colourRef"=w522) -> ()  [unwired: 9 in, 1 out]
                    n266 = call "Colour.vi"("result"="×" ("元素"), "colourRef"=w519) -> ()  [unwired: 9 in, 1 out]
                  }
                }
              }
              frame "拾取检具14" {
                n267 = call "TCP_read.vi"() -> ("元素"=w529:i8)  [unwired: 10 in, 1 out]
                n268 = Equal?(x=w529, y=i8 107) -> (x = y?=w527:bool)
                n269 = case shown="真" w527 {
                  tunnel: [w532 "放回检具14"] -> w531
                  tunnel: w530 -> [w532 _]
                  tunnel: w526 -> [_ w534]
                  frame False {
                  }
                  frame True {
                    n270 = Index Array(array=w534, index #1=14 ("索引")) -> (element #1=w538:refnum<vi>, element #2=w535:refnum<vi>)  [unwired: 1 in]
                    n271 = call "TCP_write.vi"("写入数据"=i8 108) -> ()  [unwired: 11 in]
                    n272 = call "AlarmInsert.vi"("消息名"="放回检具14" ("string_5")) -> ()  [unwired: 11 in]
                    n273 = call "Colour.vi"("result"="√" ("元素"), "colourRef"=w538) -> ()  [unwired: 9 in, 1 out]
                    n274 = call "Colour.vi"("result"="×" ("元素"), "colourRef"=w535) -> ()  [unwired: 9 in, 1 out]
                  }
                }
              }
              frame "放回检具14" {
                n275 = call "TCP_read.vi"() -> ("元素"=w545:i8)  [unwired: 10 in, 1 out]
                n276 = Equal?(x=w545, y=i8 109) -> (x = y?=w543:bool)
                n277 = case shown="真" w543 {
                  tunnel: [w548 "拾取检具15"] -> w547
                  tunnel: w546 -> [w548 _]
                  tunnel: w542 -> [_ w550]
                  frame False {
                  }
                  frame True {
                    n278 = Index Array(array=w550, index #1=15 ("索引")) -> (element #1=w554:refnum<vi>, element #2=w551:refnum<vi>)  [unwired: 1 in]
                    n279 = call "TCP_write.vi"("写入数据"=i8 110) -> ()  [unwired: 11 in]
                    n280 = call "AlarmInsert.vi"("消息名"="拾取检具15" ("string_5")) -> ()  [unwired: 11 in]
                    n281 = call "Colour.vi"("result"="√" ("元素"), "colourRef"=w554) -> ()  [unwired: 9 in, 1 out]
                    n282 = call "Colour.vi"("result"="×" ("元素"), "colourRef"=w551) -> ()  [unwired: 9 in, 1 out]
                  }
                }
              }
              frame "拾取检具15" {
                n283 = call "TCP_read.vi"() -> ("元素"=w561:i8)  [unwired: 10 in, 1 out]
                n284 = Equal?(x=w561, y=i8 111) -> (x = y?=w559:bool)
                n285 = case shown="真" w559 {
                  tunnel: [w564 "放回检具15"] -> w563
                  tunnel: w562 -> [w564 _]
                  tunnel: w558 -> [_ w566]
                  frame False {
                  }
                  frame True {
                    n286 = Index Array(array=w566, index #1=15 ("索引")) -> (element #1=w570:refnum<vi>, element #2=w567:refnum<vi>)  [unwired: 1 in]
                    n287 = call "TCP_write.vi"("写入数据"=i8 112) -> ()  [unwired: 11 in]
                    n288 = call "AlarmInsert.vi"("消息名"="放回检具15" ("string_5")) -> ()  [unwired: 11 in]
                    n289 = call "Colour.vi"("result"="√" ("元素"), "colourRef"=w570) -> ()  [unwired: 9 in, 1 out]
                    n290 = call "Colour.vi"("result"="×" ("元素"), "colourRef"=w567) -> ()  [unwired: 9 in, 1 out]
                  }
                }
              }
              frame "放回检具15" {
                n291 = call "TCP_read.vi"() -> ("元素"=w577:i8)  [unwired: 10 in, 1 out]
                n292 = Equal?(x=w577, y=i8 113) -> (x = y?=w575:bool)
                n293 = case shown="真" w575 {
                  tunnel: [w580 "判断是否合格"] -> w579
                  tunnel: w578 -> [w580 _]
                  tunnel: w574 -> [_ w582]
                  frame False {
                  }
                  frame True {
                    n294 = Index Array(array=w582, index #1=16 ("索引")) -> (element #1=w586:refnum<vi>, element #2=w583:refnum<vi>)  [unwired: 1 in]
                    n295 = call "TCP_write.vi"("写入数据"=i8 114) -> ()  [unwired: 11 in]
                    n296 = call "AlarmInsert.vi"("消息名"="判断是否合格" ("string_5")) -> ()  [unwired: 11 in]
                    n297 = call "Colour.vi"("result"="√" ("元素"), "colourRef"=w586) -> ()  [unwired: 9 in, 1 out]
                    n298 = call "Colour.vi"("result"="×" ("元素"), "colourRef"=w583) -> ()  [unwired: 9 in, 1 out]
                  }
                }
              }
              frame "判断是否合格" {
                n299 = call "TCP_read.vi"() -> ("元素"=w590:i8)  [unwired: 10 in, 1 out]
                n300 = case shown="115" w590 {
                  tunnel: [w594 w597 w607 "91"] -> w593
                  tunnel: w592 -> [w594 w597 w607 _]
                  tunnel: w591 -> [_ w599 w608 _]
                  frame Default {
                  }
                  frame 115 {
                    n301 = Index Array(array=w599, index #1=17 ("索引")) -> (element #1=w603:refnum<vi>, element #2=w600:refnum<vi>)  [unwired: 1 in]
                    n302 = global write "全局 3.vi" "总合格状态"("×" ("元素")) -> ()
                    n303 = global write "全局 3.vi" "合格判断"("×" ("元素")) -> ()
                    n304 = call "AlarmInsert.vi"("消息名"="不合格 取出工件" ("string_5")) -> ()  [unwired: 11 in]
                    n305 = call "Colour.vi"("result"="×" ("元素"), "colourRef"=w603) -> ()  [unwired: 9 in, 1 out]
                    n306 = call "Colour.vi"("result"="×" ("元素"), "colourRef"=w600) -> ()  [unwired: 9 in, 1 out]
                  }
                  frame 116 {
                    n307 = Index Array(array=w608, index #1=17 ("索引")) -> (element #1=w610:refnum<vi>, element #2=w613:refnum<vi>)  [unwired: 1 in]
                    n308 = global write "全局 3.vi" "总合格状态"("" ("元素")) -> ()
                    n309 = global write "全局 3.vi" "合格判断"("√" ("元素")) -> ()
                    n310 = call "AlarmInsert.vi"("消息名"="合格 取出工件" ("string_5")) -> ()  [unwired: 11 in]
                    n311 = call "Colour.vi"("result"="√" ("元素"), "colourRef"=w610) -> ()  [unwired: 9 in, 1 out]
                    n312 = call "Colour.vi"("result"="×" ("元素"), "colourRef"=w613) -> ()  [unwired: 9 in, 1 out]
                  }
                  frame 120 {
                  }
                }
              }
              frame "91" {
                n313 = call "TCP_read.vi"() -> ("元素"=w619:i8)  [unwired: 10 in, 1 out]
                n314 = Equal?(x=w619, y=i8 120) -> (x = y?=w617:bool)
                n315 = case shown="真" w617 {
                  tunnel: [w622 "10"] -> w621
                  tunnel: w620 -> [w622 _]
                  tunnel: w616 -> [_ w634]
                  frame False {
                  }
                  frame True {
                    n316 = global read "resultShow.vi" "Status"() -> (w626:T1)
                    n317 = global read "resultShow.vi" "countLeft"() -> (w629:refnum<vi>)
                    n318 = Unbundle By Name(w626) -> ("connectionMode"=w627:refnum<vi>)
                    n319 = Index Array(array=w634, index=18 ("索引")) -> (element=w636:refnum<vi>)
                    n320 = property class="DigNum (严格)"(reference=w629) -> (reference out=w633:refnum<vi>, "Value"=w632:u32)  [unwired: 1 in, 1 out]
                    n321 = property class="Str"(reference=w627) -> ("Value"=w625:string)  [unwired: 1 in, 2 out]
                    n322 = call "Colour.vi"("result"="√" ("元素"), "colourRef"=w636) -> ()  [unwired: 9 in, 1 out]
                    n323 = call "AlarmInsert.vi"("消息名"="完成" ("string_5")) -> ()  [unwired: 11 in]
                    n324 = Increment(x=w632) -> (x+1=w631:u32)
                    n325 = Equal?(x=w625, y="联网") -> (x = y?=w623:bool)
                    n326 = call "TCP_write.vi"("写入数据"=i8 0) -> ()  [unwired: 11 in]
                    n327 = case shown="真" w623 {
                      frame False {
                      }
                      frame True {
                        n328 = call "updateiqual.vi"() -> ()  [unwired: 11 in]
                      }
                    }
                    n329 = property class="DigNum (严格)"(reference=w633, "Value"=w631) -> ()  [unwired: 1 in, 2 out]
                  }
                }
              }
            }
            n330 = local write "stepMotor/ECU"(w24) -> ()
          }
          frame #1 {
            n331 = call "TCP_read.vi"() -> ("元素"=w645:i8)  [unwired: 10 in, 1 out]
            n332 = local read "stepMotor/ECU"() -> (w642:string)
            n333 = local read "布尔"() -> (w640:bool)
            n334 = Equal?(x=w645, y=i8 -100) -> (x = y?=w641:bool)
            n335 = Or(x=w641, y=w640) -> (x .or. y?=w639:bool)
            n336 = case shown="真" w639 {
              tunnel: [w646 w648] -> w643
              tunnel: w642 -> [w646 w647]
              frame False {
              }
              frame True {
                (unwired) "10"
                n337 = call "TCP_read.vi"() -> ("元素"=w651:i8)  [unwired: 10 in, 1 out]
                n338 = local write "布尔"(TRUE ("布尔")) -> ()
                n339 = Equal?(x=w651, y=i8 0) -> (x = y?=w650:bool)
                n340 = call "AlarmInsert.vi"("消息名"="复位中" ("string_5")) -> ()  [unwired: 11 in]
                n341 = case shown="真" w650 {
                  tunnel: [w654 "10"] -> w648
                  tunnel: w647 -> [w654 _]
                  frame False {
                  }
                  frame True {
                    n342 = local write "布尔"(FALSE ("布尔")) -> ()
                  }
                }
              }
            }
            n343 = local write "stepMotor/ECU"(w643) -> ()
          }
          frame #2 {
            n344 = global read "全局 3.vi" "stop"() -> (w657:bool)
            n345 = Wait (ms)(milliseconds to wait=u32 10 ("等待时间（毫秒）")) -> ()  [unwired: 1 out]
          }
        }
      }
    }
    frame #2 {
      n346 = global read "resultShow.vi" "runMode"() -> (w660:refnum<vi>)
      n347 = property class="Bool"(reference=w660, "Value"=FALSE ("m")) -> ()  [unwired: 1 in, 2 out]
    }
  }
  n348 = local read "毫秒计时值"() -> (w7:u32)
  n349 = Tick Count (ms)() -> (millisecond timer value=w2:u32)
  n350 = Subtract(x=w2, y=w7) -> (x-y=w3:u32)
  n351 = Divide(x=w3, y=u32 1000) -> (x/y=w5:dbl)
  n352 = Tick Count (ms)() -> (millisecond timer value=w11:u32)
  n353 = To Time Stamp(1:w5) -> (0:w6:timestamp)
  n354 = local write "毫秒计时值"(w11) -> ()
  n355 = Format Date/Time String(seconds (now)=w6) -> (date/time string=w8:string)  [unwired: 2 in]
  n356 = call "AlarmInsert.vi"("takesTime"=w8, "消息名"="完成取回工件！" ("string_5")) -> ()  [unwired: 10 in]
  n357 = call "TCP_write.vi"("写入数据"=i8 13) -> ()  [unwired: 11 in]
  n358 = call "AlarmInsert.vi"("消息名"="请放回检具1" ("string_5")) -> ()  [unwired: 11 in]
